vi "CHD_SIM_SIM_MODULE_EXECUTE.vi"(6 "FPGA_Time_Seconds":dbl=-1.0, 7 "Module Index":i32, 8 "error in (no error)":errorcluster, 9 "Battery Voltage":dbl) -> (0 "error out":errorcluster, 1 "Abs Current":dbl)   [LabVIEW 2019]
uses:
  <vilib>/Rock Robotics/WPI/ThirdParty/JAS_Junk/TrajLib/Enum/DCMOTOR_TYPES_ENUM.ctl
  CHD_SIM_SIM_Globals.vi
  <vilib>/Rock Robotics/WPI/ThirdParty/JAS_Junk/TrajLib/Trajectory_Library.lvlib
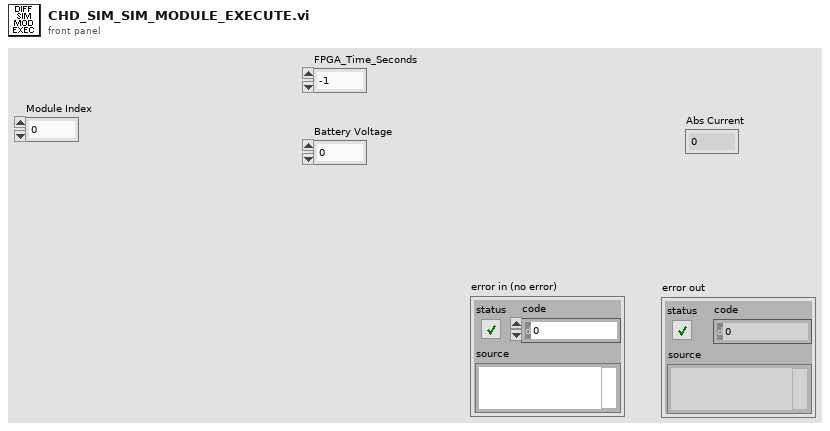
[diagram p1: front panel]
types:
  T1 = typedef "Trajectory_Library.lvlib/DCMOTOR_TYPES_ENUM.ctl" = enum16{"CIM", "AndyMark 9015", "Andy Mark RS 775 125", "Bag", "BaneBots RS 550", "BaneBots RS 775", "Falcon 500", "Mini CIM", "NEO", "NEO 550", "Romi BuiltIn", "Vex 775 Pro", "Snow Blower AM 2235A", "Bosch Seat AM 3493", "Falcon 500 FOC", "Kraken X60", "Kraken X60 FOC", "NEO Vortex", "Minion", "Kraken X44", "Kraken X44 FOC"}
  T2 = cluster{"Drive Motor Device Index":i32, "Drive Encoder Device Index":i32, "Drive DistPerzcount":dbl}[]
  T3 = cluster{"Drive Motor Device Index":i32, "Drive Encoder Device Index":i32, "Drive DistPerzcount":dbl}
  T4 = typedef "Trajectory_Library.lvlib/LINEAR_SYSTEM_ID_DCMOTOR_MODEL.ctl" = cluster{"DCMOTOR_TYPES":T1, "Num Motors":i32, "Gearing":dbl, "MOI kgm2":dbl}
  T5 = typedef "Trajectory_Library.lvlib/DCMOTOR_SIM_SIMULATION_PARAMS.ctl" = cluster{"Pos Sim Std Dev Rotations":dbl, "Vel Sim Std Dev RPM":dbl}
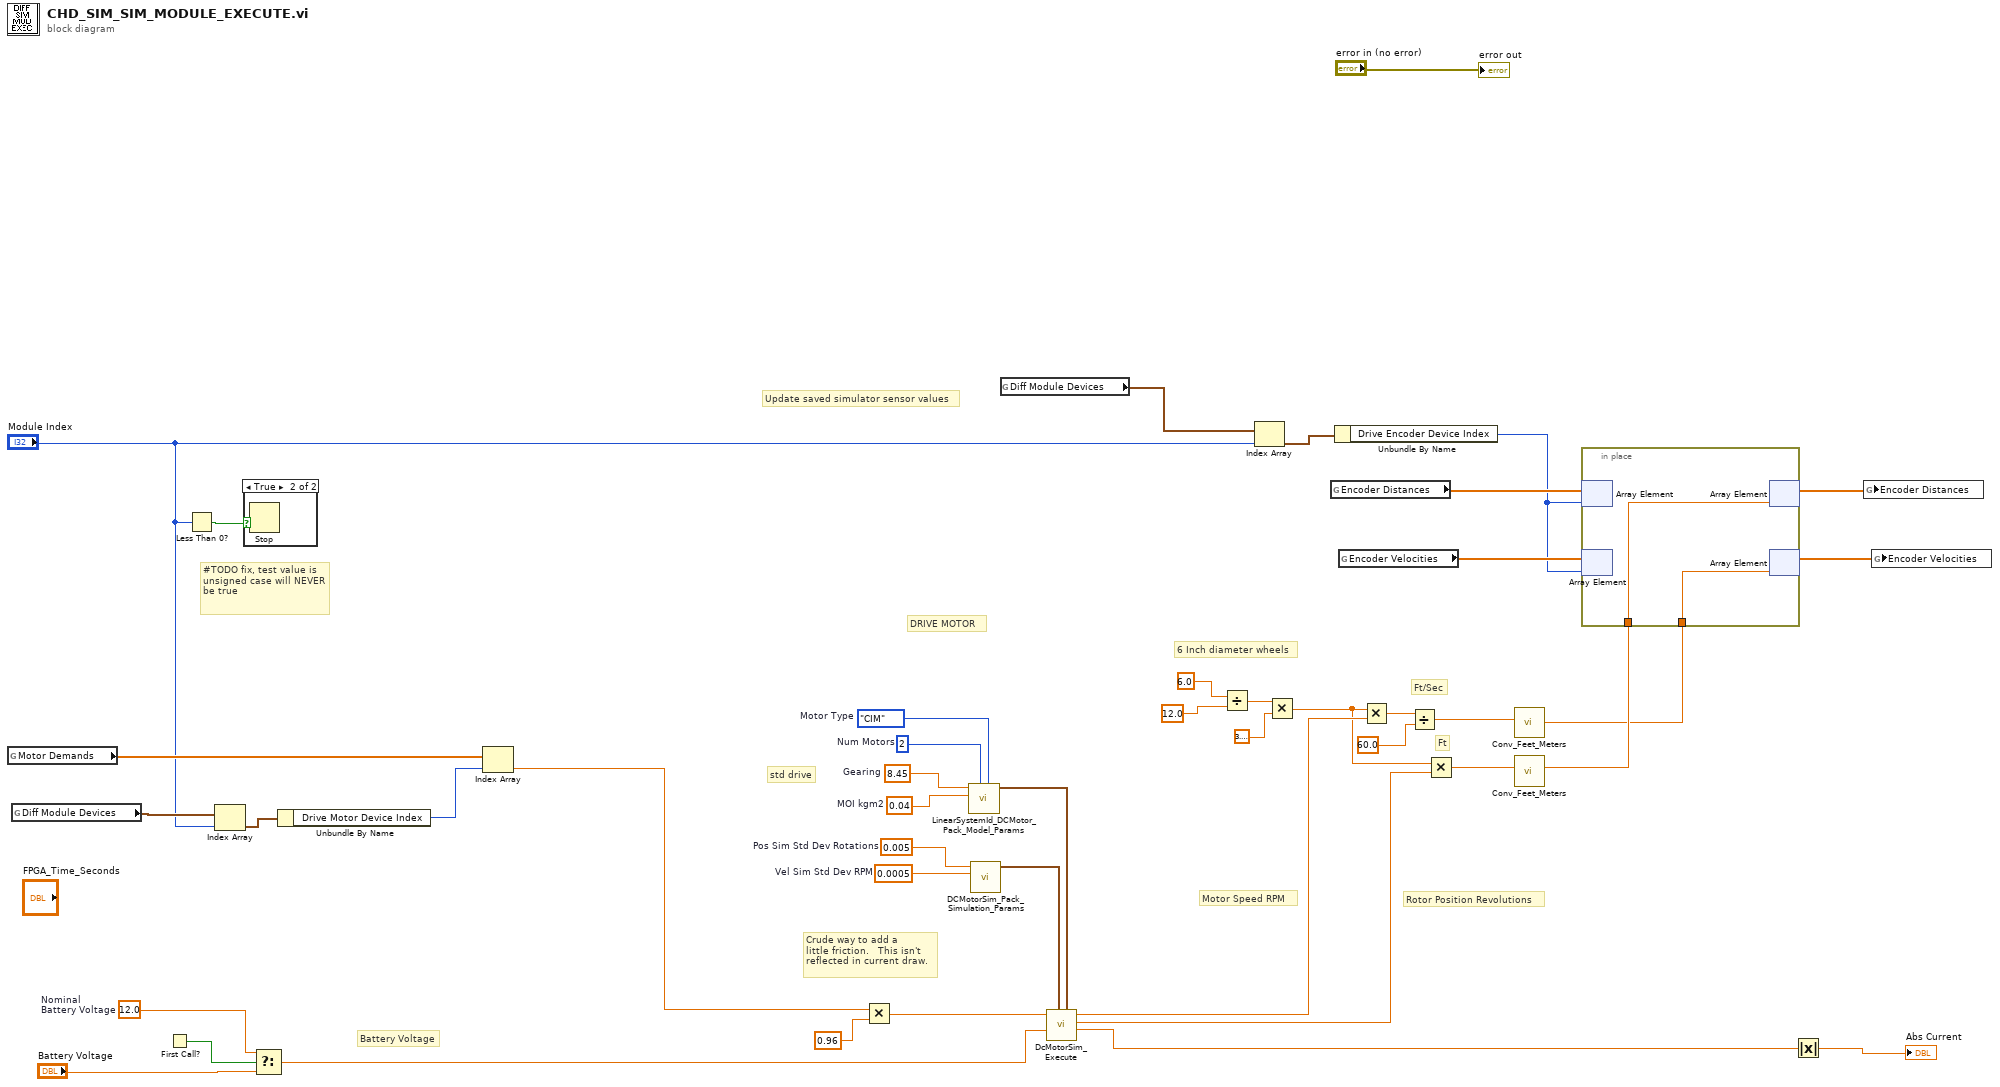
[diagram p0: block diagram]
diagram:
  w24 = 0.005  # Pos Sim Std Dev Rotations
  w25 = 0.0005  # Vel Sim Std Dev RPM
  w28 = 8.45  # Gearing
  w29 = 0.04  # MOI kgm2
  w30 = 2  # Num Motors
  w31 = DCMOTOR_TYPES_ENUM."CIM"  # Motor Type
  w22 = 12.0  # Nominal Battery Voltage
  # "Crude way to add a \nlittle friction.   This isn't\nreflected in current draw."
  # "Battery Voltage"
  # "6 Inch diameter wheels"
  # "std drive"
  # "Ft/Sec"
  # "Ft"
  # "Rotor Position Revolutions"
  # "Motor Speed RPM"
  # "DRIVE MOTOR"
  # "Update saved simulator sensor values"
  # "#TODO fix, test value is unsigned case will NEVER be true"
  n1 = global read "CHD_SIM_SIM_Globals.vi" "Motor Demands"() -> (w34:dbl[])
  n2 = global read "CHD_SIM_SIM_Globals.vi" "Diff Module Devices"() -> (w36:T2)
  n3 = First Call?() -> (First Call?: T/F=w23:bool)
  n4 = Less Than 0?(x="Module Index") -> (x < 0?=w43:bool)
  n5 = Index Array(array=w36, index="Module Index") -> (element=w35:T3)
  n6 = case shown="True" w43 {
    frame False {
    }
    frame True {
      n7 = Stop() -> ()  [unwired: 1 in]
    }
  }
  n8 = Select(t=w22, s=w23, f="Battery Voltage") -> (s? t:f=w7:dbl)
  n9 = Unbundle By Name(w35) -> ("Drive Motor Device Index"=w33:i32)
  n10 = Index Array(array=w34, index=w33) -> (element=w5:dbl)
  n11 = Multiply(x=w5, y=0.96) -> (x*y=w4:dbl)
  n12 = call <vilib>:"LinearSystemId_DCMotor_Pack_Model_Params.vi"("DCMOTOR_TYPES"=w31, "Num Motors"=w30, "MOI kgm2"=w29, "Gearing"=w28) -> ("LinearSystem_ID_DCMotor_Model"=w27:T4)  [unwired: 7 in]
  n13 = call <vilib>:"DCMotorSim_Pack_Simulation_Params.vi"("Vel Sim Std Dev RPM"=w25, "Pos Sim Std Dev Rotations"=w24) -> ("DCMOTOR_Sim_Simulation_Params"=w26:T5)  [unwired: 9 in]
  n14 = global read "CHD_SIM_SIM_Globals.vi" "Diff Module Devices"() -> (w42:T2)
  n15 = call <vilib>:"DcMotorSim_Execute.vi"("DCMotor_Model _Params"=w27, "DCMOTORSim_Simulation_Params"=w26, "Battery Voltage"=w7, "Motor Dmd (CO)"=w4) -> ("Motor Current"=w8:dbl, "Position_Rotations"=w15:dbl, "Velocity_RPM"=w17:dbl)  [unwired: 3 in, 2 out]
  n16 = Divide(x=6.0, y=12.0) -> (x/y=w19:dbl)
  n17 = Index Array(array=w42, index="Module Index") -> (element=w41:T3)
  n18 = Multiply(x=w19, y=3.141592653589793) -> (x*y=w16:dbl)
  n19 = global read "CHD_SIM_SIM_Globals.vi" "Encoder Distances"() -> (w40:dbl[])
  n20 = Unbundle By Name(w41) -> ("Drive Encoder Device Index"=w1:i32)
  n21 = global read "CHD_SIM_SIM_Globals.vi" "Encoder Velocities"() -> (w39:dbl[])
  n22 = Multiply(x=w16, y=w17) -> (x*y=w14:dbl)
  n23 = Divide(x=w14, y=60.0) -> (x/y=w12:dbl)
  n24 = Multiply(x=w16, y=w15) -> (x*y=w11:dbl)
  n25 = call <vilib>:"Conv_Feet_Meters.vi"("Feet"=w12) -> ("Meters"=w9:dbl)  [unwired: 10 in]
  n26 = call <vilib>:"Conv_Feet_Meters.vi"("Feet"=w11) -> ("Meters"=w10:dbl)  [unwired: 10 in]
  n27 = in-place {
    in-place-border: w10 -> [w45]
    in-place-border: w9 -> [w46]
    n28 = in-place-array #1(w40, w1) -> ()  [unwired: 1 out]
    n29 = in-place-array #2(w39, w1) -> ()  [unwired: 1 out]
    n30 = in-place-array #1(w45) -> (w38:dbl[])  [unwired: 1 out]
    n31 = in-place-array #2(w46) -> (w37:dbl[])  [unwired: 1 out]
  }
  n32 = Absolute Value(x=w8) -> (abs(x)=→"Abs Current":dbl)
  n33 = global write "CHD_SIM_SIM_Globals.vi" "Encoder Distances"(w38) -> ()
  n34 = global write "CHD_SIM_SIM_Globals.vi" "Encoder Velocities"(w37) -> ()
  "error out" <- "error in (no error)"
